vi "Read Temperatures Array DBL.vi"(8 "error in":errorcluster, 10 "Source":string, 11 "IRead Temperature Multichannel in":refnum<class "IRead Temperature Multichannel.lvclass">) -> (0 "error out":errorcluster, 2 "Temperatures Multichannel":dbl[][](array[numeric]), 3 "IRead Temperature Multichannel out":refnum<class "IRead Temperature Multichannel.lvclass">)   [LabVIEW 2024, in "IRead Temperature Multichannel.lvclass"]
uses:
  IRead Temperature Multichannel.lvclass
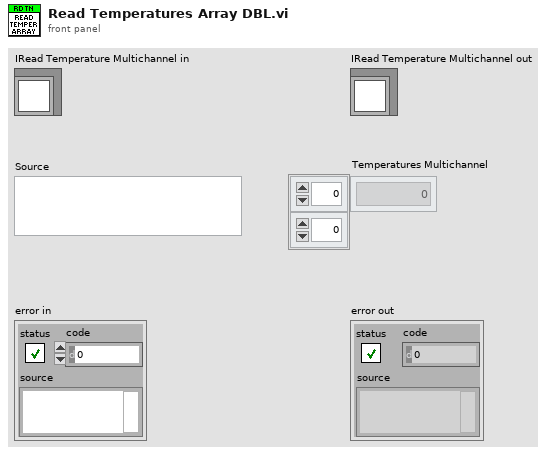
[diagram p1: front panel]
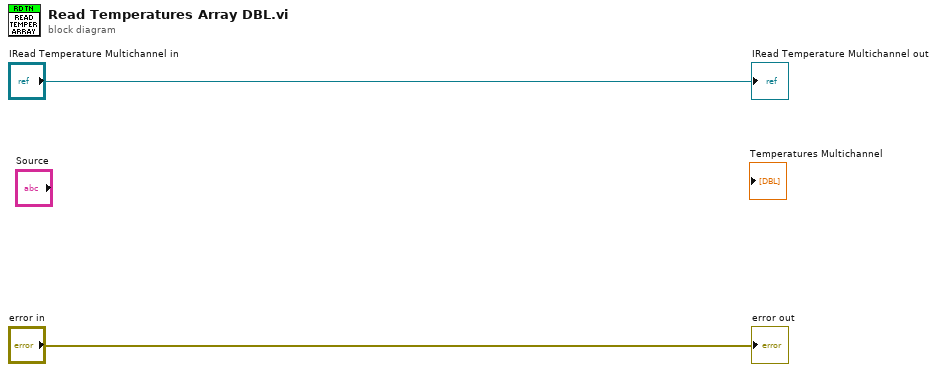
[diagram p0: block diagram]
diagram:
  "error out" <- "error in"
  "IRead Temperature Multichannel out" <- "IRead Temperature Multichannel in"
